vi "Motor Controller Set Data Rate.vi"(0 "COM port":refnum<visa-resource-name>, 5 "RS-485 addr.":u8, 7 "Data rate (Hz)":u8(ring)=14 items=["1", "2", "4", "5", "8", "10", "16", "20", "25", "32", "40", "50", "64", "80", "100", "125", "160", "200", "250", "320", "400", "500", "625", "800", "1000"], 9 "Set as power-on default":bool, 11 "Close port after action":bool) -> (4 "COM port out":refnum<visa-resource-name>, 15 "Error out":errorcluster)   [LabVIEW 2020]
uses:
  ctls/CTRL_Cmd.ctl
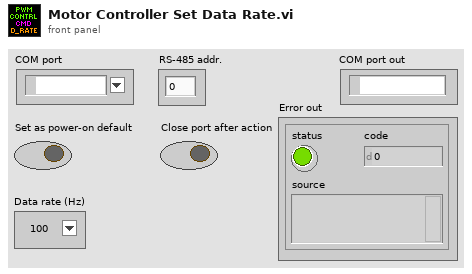
[diagram p1: front panel]
types:
  T1 = typedef "CTRL_Cmd.ctl" = string
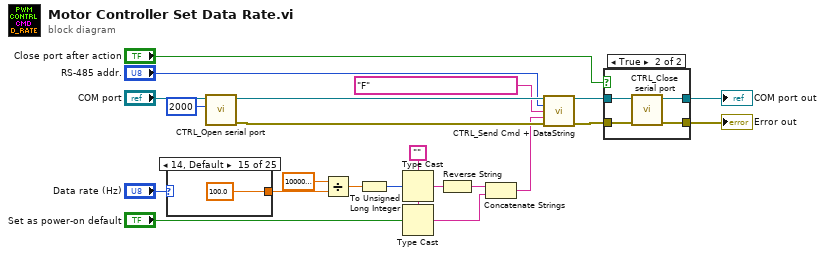
[diagram p0: block diagram]
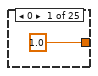
[diagram p2: hidden frame]
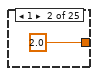
[diagram p3: hidden frame]
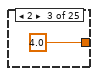
[diagram p4: hidden frame]
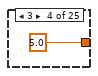
[diagram p5: hidden frame]
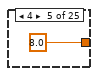
[diagram p6: hidden frame]
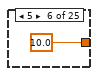
[diagram p7: hidden frame]
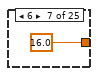
[diagram p8: hidden frame]
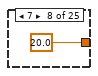
[diagram p9: hidden frame]
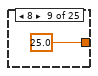
[diagram p10: hidden frame]
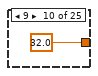
[diagram p11: hidden frame]
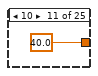
[diagram p12: hidden frame]
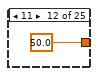
[diagram p13: hidden frame]
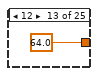
[diagram p14: hidden frame]
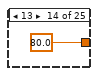
[diagram p15: hidden frame]
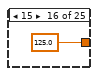
[diagram p16: hidden frame]
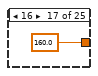
[diagram p17: hidden frame]
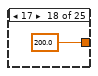
[diagram p18: hidden frame]
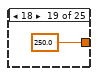
[diagram p19: hidden frame]
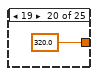
[diagram p20: hidden frame]
diagram:
  w10 = ""
  n1 = case shown="14, Default" "Data rate (Hz)" {
    tunnel: [1.0 2.0 4.0 5.0 8.0 10.0 16.0 20.0 25.0 32.0 40.0 50.0 64.0 80.0 100.0 125.0 160.0 200.0 250.0 320.0 400.0 500.0 625.0 800.0 1000.0] -> w15
    frame 0 {
    }
    frame 1 {
    }
    frame 2 {
    }
    frame 3 {
    }
    frame 4 {
    }
    frame 5 {
    }
    frame 6 {
    }
    frame 7 {
    }
    frame 8 {
    }
    frame 9 {
    }
    frame 10 {
    }
    frame 11 {
    }
    frame 12 {
    }
    frame 13 {
    }
    frame 14, Default {
    }
    frame 15 {
    }
    frame 16 {
    }
    frame 17 {
    }
    frame 18 {
    }
    frame 19 {
    }
    frame 20 {
    }
    frame 21 {
    }
    frame 22 {
    }
    frame 23 {
    }
    frame 24 {
    }
  }
  n2 = call "CTRL_Open serial port.vi"("timeout (ms)"=u32 2000, "VISA resource name"="COM port") -> ("Error out"=w19:errorcluster, "VISA resource name out"=w20:refnum<visa-resource-name>)  [unwired: 8 in]
  n3 = Divide(x=1000000.0, y=w15) -> (x/y=w9:dbl)
  n4 = To Unsigned Long Integer(number=w9) -> (unsigned 32bit integer=w2:u32)
  n5 = Type Cast(type=w10, x=w2) -> (*(type *) &x=w11:string)
  n6 = Type Cast(type=w10, x="Set as power-on default") -> (*(type *) &x=w6:string)
  n7 = Reverse String(1:w11) -> (0:w7:string)
  n8 = Concatenate Strings(w7, w6) -> (w5:string)
  n9 = call "CTRL_Send Cmd + DataString.vi"("Port"=w20, "RS-485 addr."="RS-485 addr.", "Cmd"=T1 "F", "DataString"=w5, "Error In"=w19) -> ("Port out"=w18:refnum<visa-resource-name>, "Error Out"=w4:errorcluster)  [unwired: 9 in]
  n10 = case shown="True" "Close port after action" {
    tunnel: [w49 w52] -> w17
    tunnel: w18 -> [w48 w50]
    tunnel: w4 -> [w49 w51]
    tunnel: [w48 w50] -> w1
    frame False {
    }
    frame True {
      n11 = call "CTRL_Close serial port.vi"("Error in"=w51, "VISA resource name"=w50) -> ("Error out"=w52:errorcluster)  [unwired: 9 in]
    }
  }
  "Error out" <- w17
  "COM port out" <- w1
